vi "InitProduct.vi"(0 "SENSOR":T1={"hSENSOR"=268435457, "hASIC_T1"=268435458, "hASIC_T2"=268435460, "hASIC_P"=268435459, "hASIC_S"=268435457}, 11 "error in (no error)":errorcluster caption="错误输入（无错误）") -> (6 "hSENSOR out":i32, 15 "error out":errorcluster caption="错误输出")   [LabVIEW 2020]
doc: "该模板用于创建子VI。"
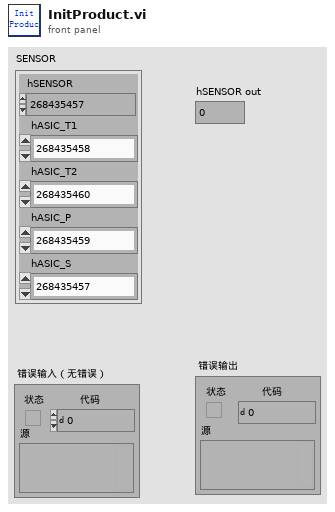
[diagram p1: front panel]
types:
  T1 = cluster{"hSENSOR":i32, "hASIC_T1":i32, "hASIC_T2":i32, "hASIC_P":i32, "hASIC_S":i32}
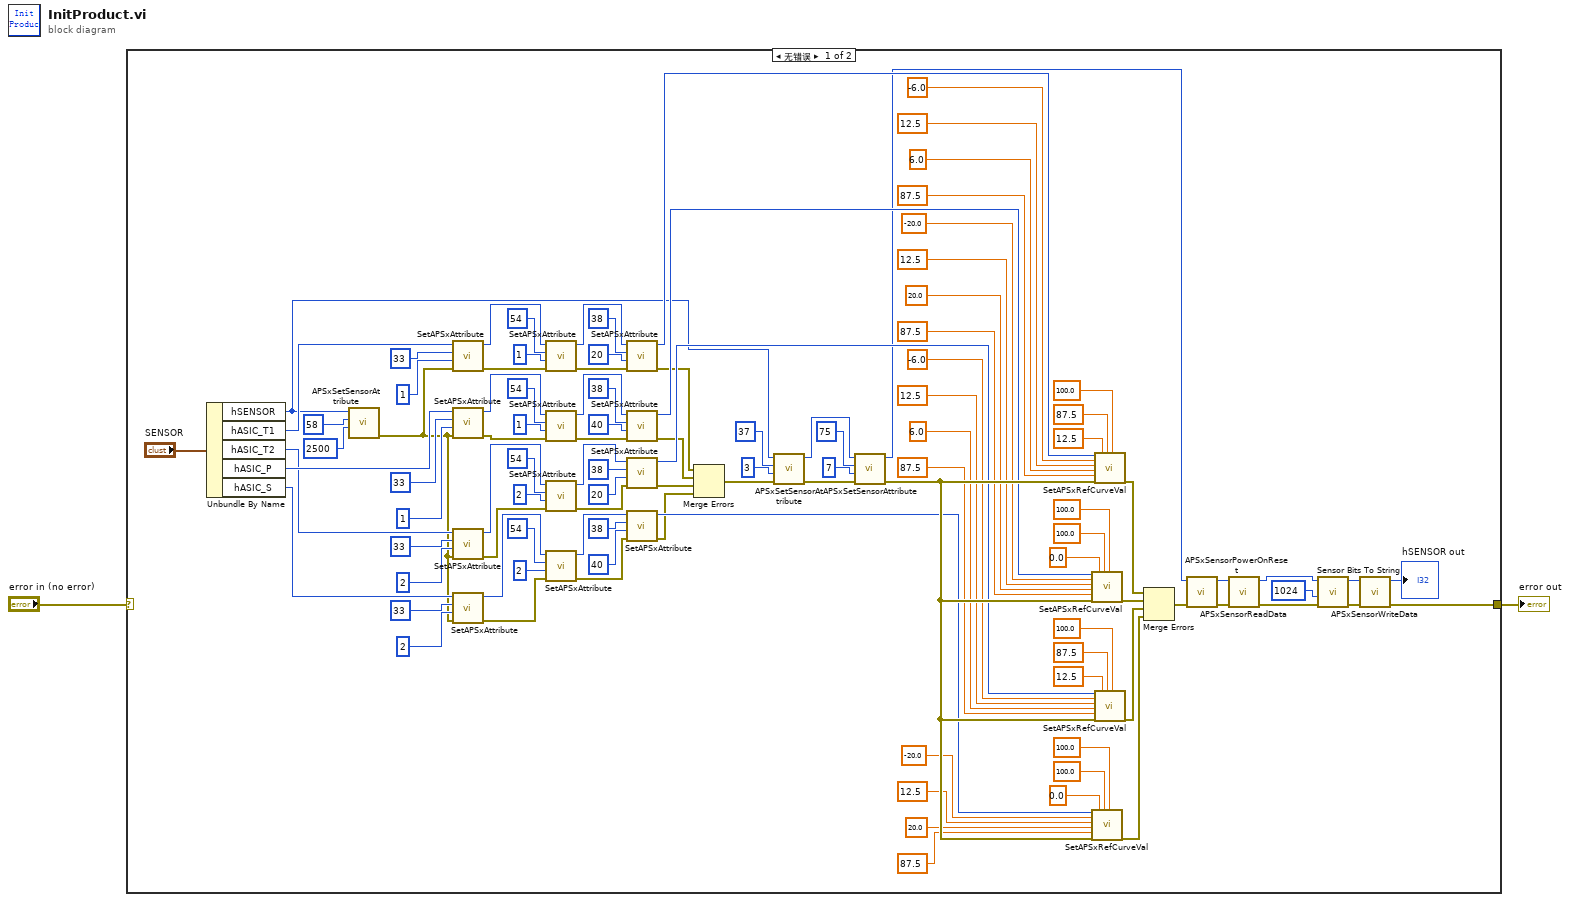
[diagram p0: block diagram]
diagram:
  n1 = case shown="无错误" "error in (no error)" {
    selector: "error in (no error)" -> [_ w111]
    tunnel: [w57 w111] -> w1
    frame No Error {
      n2 = Unbundle By Name("SENSOR") -> ("hSENSOR"=w43:i32, "hASIC_T1"=w55:i32, "hASIC_T2"=w53:i32, "hASIC_P"=w54:i32, "hASIC_S"=w52:i32)
      n3 = call "APSxSetSensorAttribute.vi"("Param2"=2500, "Param1"=58, "hSENSOR"=w43) -> ("error out"=w40:errorcluster)  [unwired: 6 in, 2 out]
      n4 = call "SetAPSxAttribute.vi"("error in (no error)"=w40, "Param2"=1, "Param1"=33, "hASIC"=w55) -> ("error out"=w82:errorcluster, "hASIC out"=w84:i32)  [unwired: 5 in, 1 out]
      n5 = call "SetAPSxAttribute.vi"("error in (no error)"=w40, "Param2"=1, "Param1"=33, "hASIC"=w54) -> ("error out"=w81:errorcluster, "hASIC out"=w83:i32)  [unwired: 5 in, 1 out]
      n6 = call "SetAPSxAttribute.vi"("error in (no error)"=w40, "Param2"=2, "Param1"=33, "hASIC"=w53) -> ("error out"=w79:errorcluster, "hASIC out"=w80:i32)  [unwired: 5 in, 1 out]
      n7 = call "SetAPSxAttribute.vi"("error in (no error)"=w40, "Param2"=2, "Param1"=33, "hASIC"=w52) -> ("error out"=w77:errorcluster, "hASIC out"=w78:i32)  [unwired: 5 in, 1 out]
      n8 = call "SetAPSxAttribute.vi"("error in (no error)"=w82, "Param2"=1, "Param1"=54, "hASIC"=w84) -> ("error out"=w50:errorcluster, "hASIC out"=w51:i32)  [unwired: 5 in, 1 out]
      n9 = call "SetAPSxAttribute.vi"("error in (no error)"=w81, "Param2"=1, "Param1"=54, "hASIC"=w83) -> ("error out"=w48:errorcluster, "hASIC out"=w49:i32)  [unwired: 5 in, 1 out]
      n10 = call "SetAPSxAttribute.vi"("error in (no error)"=w79, "Param2"=2, "Param1"=54, "hASIC"=w80) -> ("error out"=w46:errorcluster, "hASIC out"=w47:i32)  [unwired: 5 in, 1 out]
      n11 = call "SetAPSxAttribute.vi"("error in (no error)"=w77, "Param2"=2, "Param1"=54, "hASIC"=w78) -> ("error out"=w44:errorcluster, "hASIC out"=w45:i32)  [unwired: 5 in, 1 out]
      n12 = call "SetAPSxAttribute.vi"("error in (no error)"=w50, "Param2"=20, "Param1"=38, "hASIC"=w51) -> ("error out"=w66:errorcluster, "hASIC out"=w101:i32)  [unwired: 5 in, 1 out]
      n13 = call "SetAPSxAttribute.vi"("error in (no error)"=w48, "Param2"=40, "Param1"=38, "hASIC"=w49) -> ("error out"=w65:errorcluster, "hASIC out"=w103:i32)  [unwired: 5 in, 1 out]
      n14 = call "SetAPSxAttribute.vi"("error in (no error)"=w46, "Param2"=20, "Param1"=38, "hASIC"=w47) -> ("error out"=w64:errorcluster, "hASIC out"=w104:i32)  [unwired: 5 in, 1 out]
      n15 = call "SetAPSxAttribute.vi"("error in (no error)"=w44, "Param2"=40, "Param1"=38, "hASIC"=w45) -> ("error out"=w63:errorcluster, "hASIC out"=w105:i32)  [unwired: 5 in, 1 out]
      n16 = Merge Errors(w66, w65, w64, w63) -> (w62:errorcluster)
      n17 = call "APSxSetSensorAttribute.vi"("error in (no error)"=w62, "Param2"=3, "Param1"=37, "hSENSOR"=w43) -> ("error out"=w59:errorcluster, "hSENSOR out"=w102:i32)  [unwired: 5 in, 1 out]
      n18 = call "APSxSetSensorAttribute.vi"("error in (no error)"=w59, "Param2"=7, "Param1"=75, "hSENSOR"=w102) -> ("error out"=w106:errorcluster, "hSENSOR out"=w58:i32)  [unwired: 5 in, 1 out]
      n19 = call "SetAPSxRefCurveVal.vi"("hASIC"=w103, "LeftX"=-20.0, "LeftY"=12.5, "RightX"=20.0, "RightY"=87.5, "error in (no error)"=w106, "LowerLimit"=0.0, "UpperLimit"=100.0, "yScale"=100.0) -> ("error out"=w108:errorcluster)  [unwired: 8 in, 2 out]
      n20 = call "SetAPSxRefCurveVal.vi"("hASIC"=w105, "LeftX"=-20.0, "LeftY"=12.5, "RightX"=20.0, "RightY"=87.5, "error in (no error)"=w106, "LowerLimit"=0.0, "UpperLimit"=100.0, "yScale"=100.0) -> ("error out"=w110:errorcluster)  [unwired: 8 in, 2 out]
      n21 = call "SetAPSxRefCurveVal.vi"("hASIC"=w101, "LeftX"=-6.0, "LeftY"=12.5, "RightX"=6.0, "RightY"=87.5, "error in (no error)"=w106, "LowerLimit"=12.5, "UpperLimit"=87.5, "yScale"=100.0) -> ("error out"=w107:errorcluster)  [unwired: 8 in, 2 out]
      n22 = call "SetAPSxRefCurveVal.vi"("hASIC"=w104, "LeftX"=-6.0, "LeftY"=12.5, "RightX"=6.0, "RightY"=87.5, "error in (no error)"=w106, "LowerLimit"=12.5, "UpperLimit"=87.5, "yScale"=100.0) -> ("error out"=w109:errorcluster)  [unwired: 8 in, 2 out]
      n23 = Merge Errors(w107, w108, w109, w110) -> (w11:errorcluster)
      n24 = call "APSxSensorPowerOnReset.vi"("error in (no error)"=w11, "hSENSOR"=w58) -> ("error out"=w8:errorcluster, "hSENSOR out"=w9:i32)  [unwired: 7 in, 1 out]
      n25 = call "APSxSensorReadData.vi"("error in (no error)"=w8, "hSENSOR"=w9) -> ("error out"=w7:errorcluster, "hSENSOR out"=w10:i32)  [unwired: 7 in, 1 out]
      n26 = call "Sensor Bits To String.vi"("error in (no error)"=w7, "BitBufferSize"=1024, "sensorHandle"=w10) -> ("error out"=w3:errorcluster, "function return"=w4:i32)  [unwired: 6 in, 1 out]
      n27 = call "APSxSensorWriteData.vi"("error in (no error)"=w3, "hSENSOR"=w4) -> ("error out"=w57:errorcluster, "hSENSOR out"=→"hSENSOR out":i32)  [unwired: 7 in, 1 out]
    }
    frame Error {
    }
  }
  "error out" <- w1
